vi "M Solar cells.vi"(11 "EV3 in":T1) -> (3 "EV3 out":T1)   [LabVIEW 2016]
uses:
  <vilib>/NXT/Subs/LVHSConnector.ctl
  <vilib>/NXT/LegoClasses/BrickReference/BrickReference.lvclass
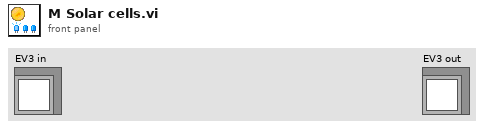
[diagram p1: front panel]
types:
  T1 = typedef "LVHSConnector.ctl" = refnum<class "BrickReference.lvclass">
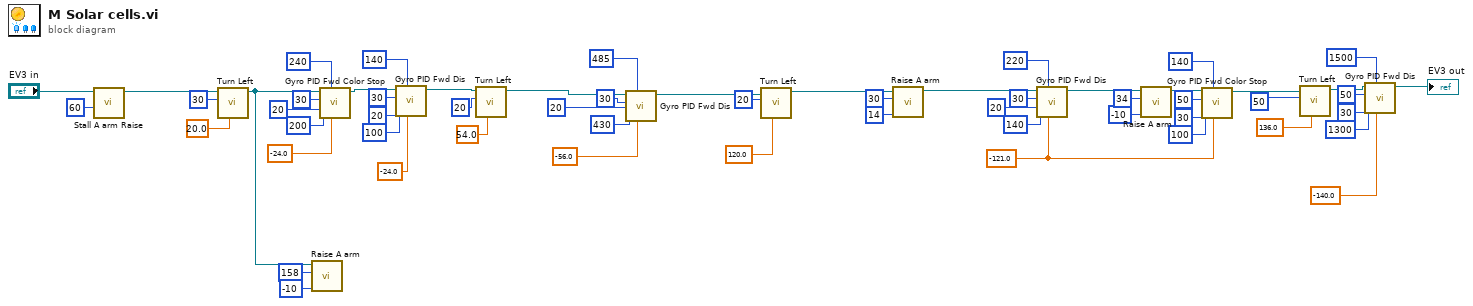
[diagram p0: block diagram]
diagram:
  w8 = sgl -121.0 ("Target angle")
  n1 = call "Stall A arm Raise.vi"("Power"=i8 60, "NXT/EV3"="EV3 in") -> ("NXT/EV3"=w27:T1)  [unwired: 9 in]
  n2 = call "Turn Left.vi"("Turning angle"=sgl 20.0, "Motor B (right)"=i8 30, "EV3 in"=w27) -> ("EV3 out"=w26:T1)  [unwired: 8 in]
  n3 = call "Raise A arm.vi"("Power"=i8 -10, "Rotation"=158, "EV3 in"=w26) -> ()  [unwired: 8 in, 1 out]
  n4 = call "Gyro PID Fwd Color Stop.vi"("Target angle"=sgl -24.0, "Threshold to Color"=240, "Threshold to slow"=200, "Min. speed"=20, "Max. speed"=30, "EV3 in"=w26) -> ("EV3 out"=w22:T1)  [unwired: 5 in]
  n5 = call "Gyro PID Fwd Dis.vi"("Target angle"=sgl -24.0, "Threshold to stop"=140, "Threshold to slow"=100, "Min. speed"=20, "Max. speed"=30, "EV3 in"=w22) -> ("EV3 out"=w23:T1)  [unwired: 5 in]
  n6 = call "Turn Left.vi"("Turning angle"=sgl 54.0, "Motor B (right)"=i8 20, "EV3 in"=w23) -> ("EV3 out"=w50:T1)  [unwired: 8 in]
  n7 = call "Gyro PID Fwd Dis.vi"("Target angle"=sgl -56.0, "Threshold to stop"=485, "Threshold to slow"=430, "Min. speed"=20, "Max. speed"=30, "EV3 in"=w50) -> ("EV3 out"=w40:T1)  [unwired: 5 in]
  n8 = call "Turn Left.vi"("Turning angle"=sgl 120.0, "Motor B (right)"=i8 20, "EV3 in"=w40) -> ("EV3 out"=w37:T1)  [unwired: 8 in]
  n9 = call "Raise A arm.vi"("Power"=i8 14, "Rotation"=30, "EV3 in"=w37) -> ("EV3 out"=w32:T1)  [unwired: 8 in]
  n10 = call "Gyro PID Fwd Dis.vi"("Target angle"=w8, "Threshold to stop"=220, "Threshold to slow"=140, "Min. speed"=20, "Max. speed"=30, "EV3 in"=w32) -> ("EV3 out"=w28:T1)  [unwired: 5 in]
  n11 = call "Raise A arm.vi"("Power"=i8 -10, "Rotation"=34, "EV3 in"=w28) -> ("EV3 out"=w14:T1)  [unwired: 8 in]
  n12 = call "Gyro PID Fwd Color Stop.vi"("Target angle"=w8, "Threshold to Color"=140, "Threshold to slow"=100, "Min. speed"=30, "Max. speed"=50, "EV3 in"=w14) -> ("EV3 out"=w13:T1)  [unwired: 5 in]
  n13 = call "Turn Left.vi"("Turning angle"=sgl 136.0, "Motor B (right)"=i8 50, "EV3 in"=w13) -> ("EV3 out"=w7:T1)  [unwired: 8 in]
  n14 = call "Gyro PID Fwd Dis.vi"("Target angle"=sgl -140.0, "Threshold to stop"=1500, "Threshold to slow"=1300, "Min. speed"=30, "Max. speed"=50, "EV3 in"=w7) -> ("EV3 out"=→"EV3 out":T1)  [unwired: 5 in]
